vi "BME_DG_CalibrateGroup_from_File.vi"(8 "error in (no error)":errorcluster, 10 "p_MasterOrSlave":T1[](array[typedef]), 11 "Path":path) -> (0 "error out":errorcluster, 3 "return code":i32)   [LabVIEW 2009]
uses:
  BME_DG_MasterOrSlave.ctl
  BME DLL/DelayGenerator.dll
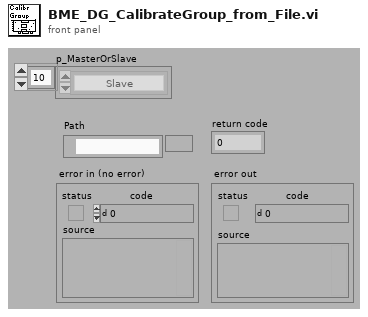
[diagram p1: front panel]
types:
  T1 = typedef "BME_DG_MasterOrSlave.ctl" = enum16{"Unknown", "Master", "Slave"}
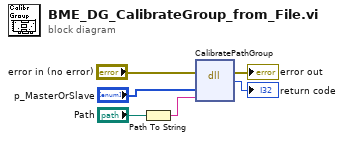
[diagram p0: block diagram]
diagram:
  n1 = Path To String(path="Path") -> (string=w2:string)
  n2 = dll-call lib="C:/Dokumente und Einstellungen/A2.5/Desktop/POLARIS BME DG/BME DLL/DelayGenerator.dll" fn="CalibratePathGroup" label="Release_DG_Data"(error in="error in (no error)", "p_MasterOrSlave"="p_MasterOrSlave", "Path"=w2) -> (error out=→"error out":errorcluster, "return type"=→"return code":i32)  [unwired: 4 in, 1 out]
